vi "Set External Control.vi"(8 "error in (no error)":errorcluster, 10 "External Control":bool, 11 "VISA session":refnum<visa-resource-name>) -> (0 "error out":errorcluster, 3 "dup VISA session":refnum<visa-resource-name>)   [LabVIEW 2011, in "Magna PSU.lvlib"]
uses:
  Magna PSU.lvlib
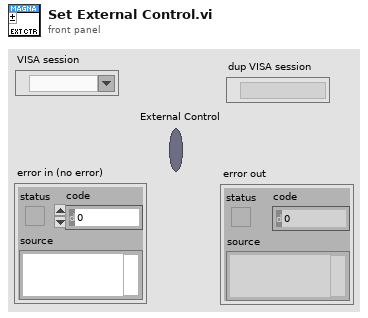
[diagram p1: front panel]
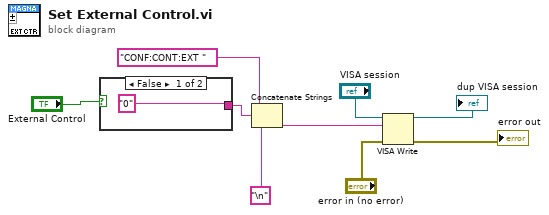
[diagram p0: block diagram]
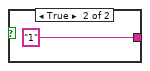
[diagram p2: hidden frame]
diagram:
  n1 = case shown="False" "External Control" {
    tunnel: ["0" "1"] -> w6
    frame False {
    }
    frame True {
    }
  }
  n2 = Concatenate Strings("CONF:CONT:EXT ", w6, "\n") -> (w8:string)
  n3 = VISA Write(VISA resource name="VISA session", write buffer=w8, error in (no error)="error in (no error)") -> (VISA resource name out=→"dup VISA session":refnum<visa-resource-name>, error out=→"error out":errorcluster)  [unwired: 1 out]
